vi "API Init Module.vi"(8 "Error In":errorcluster, 11 "GUI Object Refs":T1) -> (0 "Error Out":errorcluster)   [LabVIEW 2022 SP3]
doc: "Enqueues the \"Init Module\" command."
uses:
  GUI Object Refs (cluster).ctl
  Command.ctl
panel:
  # "Development\ncontrols/indicators useful for development and testing, but which are not outputs of the VI"
  # "Input\nInputs to the VI"
  # "Output\nOutputs of the VI"
  # "Description\n\nBlank VI with error handling case. \n\nSummarize the use of this VI in this space."
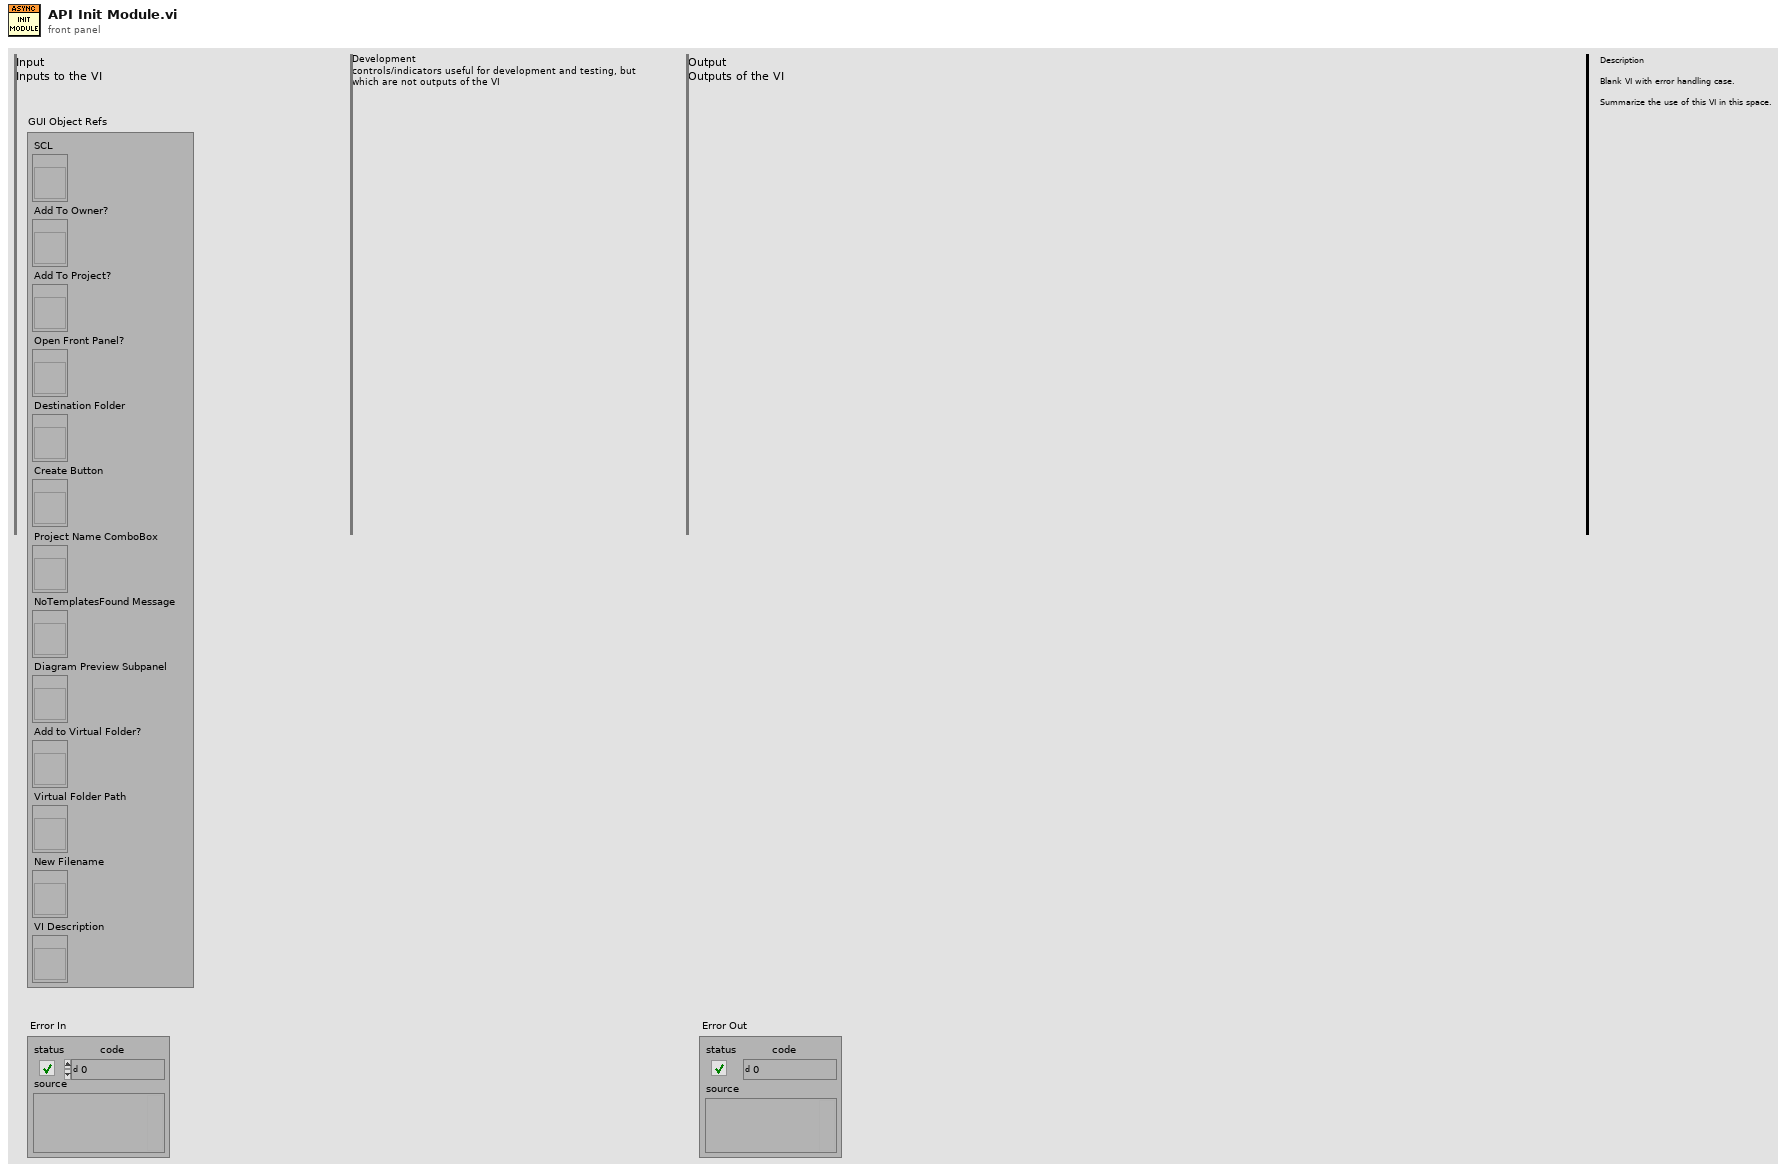
[diagram p1: front panel]
types:
  T1 = typedef "GUI Object Refs (cluster).ctl" = cluster{"SCL":refnum<vi>, "Add To Owner?":refnum<vi>, "Add To Project?":refnum<vi>, "Open Front Panel?":refnum<vi>, "Destination Folder":refnum<vi>, "Create Button":refnum<vi>, "Project Name ComboBox":refnum<vi>, "NoTemplatesFound Message":refnum<vi>, "Diagram Preview Subpanel":refnum<vi>, "Add to Virtual Folder?":refnum<vi>, "Virtual Folder Path":refnum<vi>, "New Filename":refnum<vi>, "VI Description":refnum<vi>}
  T2 = typedef "Command.ctl" = enum16{"Init Module", "Close Module", "Local Error Handler", "Init Tickboxes", "Command 2 (replace me)", "Command 3 (replace me)"}
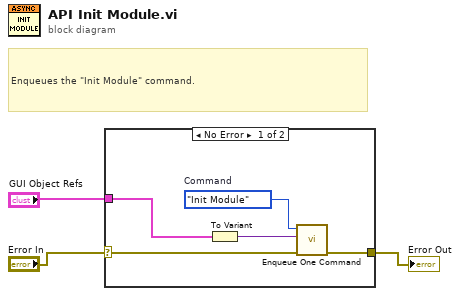
[diagram p0: block diagram]
diagram:
  # "Enqueues the \"Init Module\" command."
  n1 = case shown="No Error" "Error In" {
    selector: "Error In" -> [w7 w9]
    tunnel: [w6 w9] -> w2
    tunnel: "GUI Object Refs" -> [w5 _]
    frame No Error {
      w8 = Command."Init Module"  # Command
      n2 = To Variant(anything=w5) -> (Variant=w4:variant)
      n3 = call "Enqueue One Command.vi"("error in (no error)"=w7, "Data"=w4, "Command"=w8) -> ("error out"=w6:errorcluster)  [unwired: 8 in]
    }
    frame Error {
    }
  }
  "Error Out" <- w2
